vi "VolumeScanWizard Popup.vi"(10 "Row":i32, 11 "Axes":string[](array[string])) -> (2 "Selection":u16, 3 "Cancelled":bool)   [LabVIEW 2015]
panel:
  in  "Cancel Button":bool
  in  "OK Button":bool
  out "Message":string
  in  "Axis names":u16(ring) items=["A", "B"]
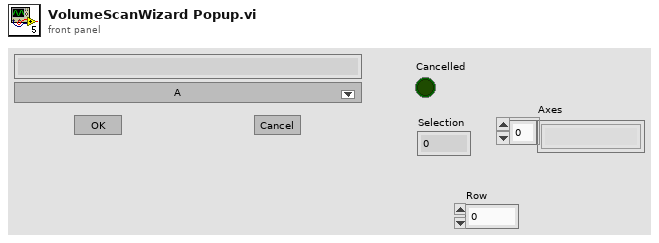
[diagram p1: front panel]
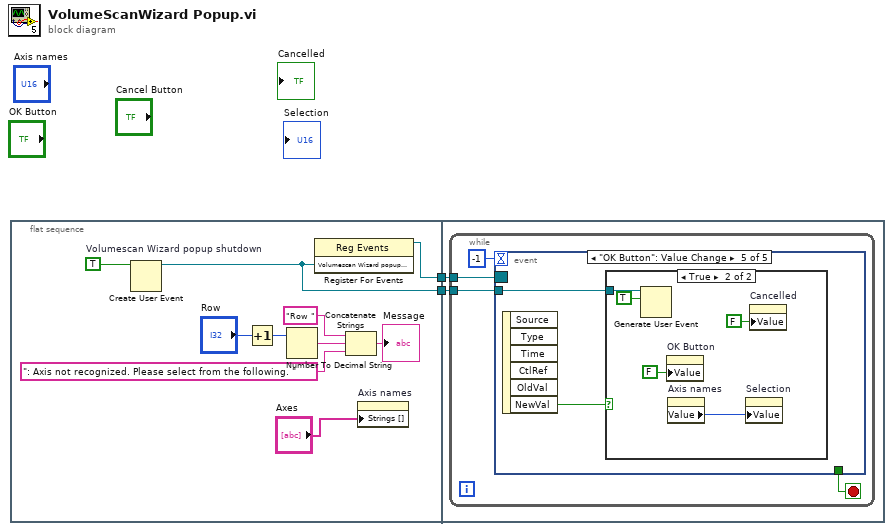
[diagram p0: block diagram]
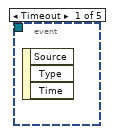
[diagram p2: hidden frame]
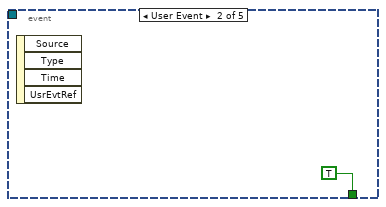
[diagram p3: hidden frame]
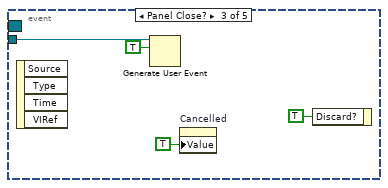
[diagram p4: hidden frame]
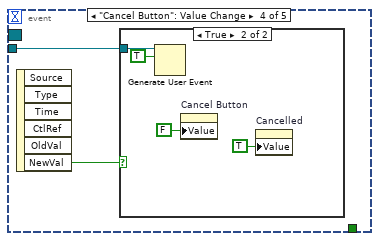
[diagram p5: hidden frame]
diagram:
  n1 = flat-sequence {
    tunnel: [w7] -> w2
    tunnel: [w6] -> w1
    tunnel: w2 -> [w14]
    tunnel: w1 -> [w13]
    frame #0 {
      w8 = TRUE  # Volumescan Wizard popup shutdown
      n2 = Create User Event(user event datatype=w8) -> (user event=w6:refnum<user-event>)  [unwired: 1 in, 1 out]
      n3 = Increment(x="Row") -> (x+1=w3:i32)
      n4 = Number To Decimal String(number=w3) -> (decimal integer string=w11:string)  [unwired: 1 in]
      n5 = register-events(w6) -> (reference out=w7:refnum<event-registration>)  [unwired: 2 in, 1 out]
      n6 = Concatenate Strings("Row ", w11, ": Axis not recognized. Please select from the following. ") -> (→"Message":string)
      n7 = property on="Axis names" class="Ring (strict)"("Strings []"="Axes") -> ()  [unwired: 2 in, 2 out]
    }
    frame #1 {
      n8 = while {
        tunnel: w14 -> [w17]
        tunnel: w13 -> [w16]
        stop <- w15 stop-if-true
        n9 = event shown="[4] \"OK Button\": Value Change" {
          selector: w17 -> [_ _ _ _ _]
          dyn-events: _ -> [_ _ _ _ _]
          timeout: -1 -> [_ _ _ _ _]
          tunnel: w16 -> [_ _ w22 w25 w31]
          tunnel: [_ TRUE _ _ _] -> w15
          event Timeout {
            n10 = event-data() -> ()  [unwired: 1 in, 3 out]
          }
          event User Event {
            n11 = event-data() -> ()  [unwired: 1 in, 4 out]
          }
          event Panel Close? {
            n12 = event-data() -> ()  [unwired: 1 in, 4 out]
            n13 = Generate User Event(user event=w22, event data cluster=TRUE ("event data")) -> ()  [unwired: 2 in, 2 out]
            n14 = property on="Cancelled" class="Bool (strict)"("Value"=TRUE ("Cancelled")) -> ()  [unwired: 2 in, 2 out]
            n15 = event-data("Discard?"=TRUE) -> ()  [unwired: 1 in, 1 out]
          }
          event "Cancel Button": Value Change {
            n16 = event-data() -> ("NewVal"=w24:bool)  [unwired: 1 in, 5 out]
            n17 = case shown="True" w24 {
              tunnel: w25 -> [_ w29]
              frame False {
              }
              frame True {
                n18 = Generate User Event(user event=w29, event data cluster=TRUE ("event data")) -> ()  [unwired: 2 in, 2 out]
                n19 = property on="Cancel Button" class="Bool (strict)"("Value"=FALSE ("Cancel Button")) -> ()  [unwired: 2 in, 2 out]
                n20 = property on="Cancelled" class="Bool (strict)"("Value"=TRUE ("Cancelled")) -> ()  [unwired: 2 in, 2 out]
              }
            }
          }
          event "OK Button": Value Change {
            n21 = event-data() -> ("NewVal"=w30:bool)  [unwired: 1 in, 5 out]
            n22 = case shown="True" w30 {
              tunnel: w31 -> [_ w36]
              frame False {
              }
              frame True {
                n23 = Generate User Event(user event=w36, event data cluster=TRUE ("event data")) -> ()  [unwired: 2 in, 2 out]
                n24 = property on="OK Button" class="Bool (strict)"("Value"=FALSE ("Cancel Button")) -> ()  [unwired: 2 in, 2 out]
                n25 = property on="Axis names" class="Ring (strict)"() -> ("Value"=w32:u16)  [unwired: 2 in, 2 out]
                n26 = property on="Selection" class="DigNum (strict)"("Value"=w32) -> ()  [unwired: 2 in, 2 out]
                n27 = property on="Cancelled" class="Bool (strict)"("Value"=FALSE ("Cancelled")) -> ()  [unwired: 2 in, 2 out]
              }
            }
          }
        }
      }
    }
  }
